vi "mcl sort test.vi"() -> ()   [LabVIEW 2010]
panel:
  in  "Stop":bool
  in  "Multicolumn Listbox":i32(listbox)
  in  "Table of Shots":string[][](table) caption="Shot Table"
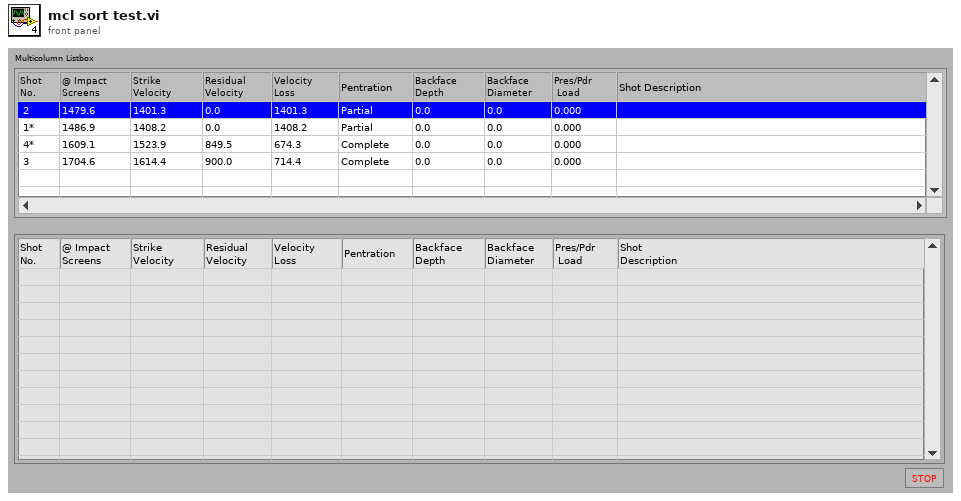
[diagram p1: front panel]
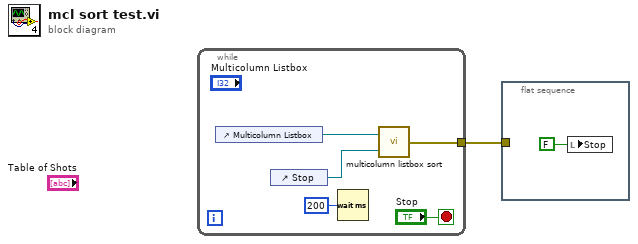
[diagram p0: block diagram]
diagram:
  n1 = while {
    tunnel: [w2] -> w1
    stop <- "Stop" stop-if-true
    n2 = control-ref of="Multicolumn Listbox"() -> (w6:refnum<vi>)
    n3 = control-ref of="Stop"() -> (w5:refnum<vi>)
    n4 = Wait (ms)(milliseconds to wait=u32 200) -> ()  [unwired: 1 out]
    n5 = call "multicolumn listbox sort.vi"("Bool Refnum"=w5, "MCListbox Refnum"=w6) -> ("error out"=w2:errorcluster)
  }
  n6 = flat-sequence {
    tunnel: w1 -> [_]
    frame #0 {
      n7 = local write "Stop"(FALSE ("Stop")) -> ()
    }
  }
